vi "Constructor.vi"() -> ()   [LabVIEW 2015, in "IO Class.lvclass"]
uses:
  IO Class.lvclass
  Signal Settings.ctl
  Configuration.ctl
  Digital Indicator/Digital Indicator.lvclass
  Digital Control/Digital Control.lvclass
  Numeric Indicator/Numeric Indicator.lvclass
  Numeric Control/Numeric Control.lvclass
  FPGA Addon Input/FPGA Addon Input.lvclass
  FPGA Addon Output/FPGA Addon Output.lvclass
  IO Class.lvclass/IO Class.ctl
  EST Digital Event/Digital Event.lvclass
  EST Output/EST Output.lvclass
  EST Knock Sensor/EST Knock Sensor.lvclass
panel:
  out "IO Class.lvclass":refnum<class "IO Class.lvclass">
  out "error out":errorcluster
  in  "error in (no error)":errorcluster
  in  "Signal Settings":T1
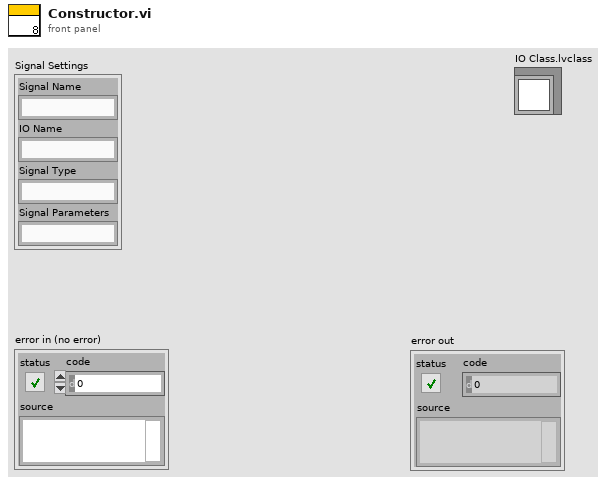
[diagram p1: front panel]
types:
  T1 = typedef "Signal Settings.ctl" = cluster{"Signal Name":string, "IO Name":string, "Signal Type":string, "Signal Parameters":string}
  T2 = typedef "Configuration.ctl" = cluster{"Classification":string, "Direction":string, "Type":string}
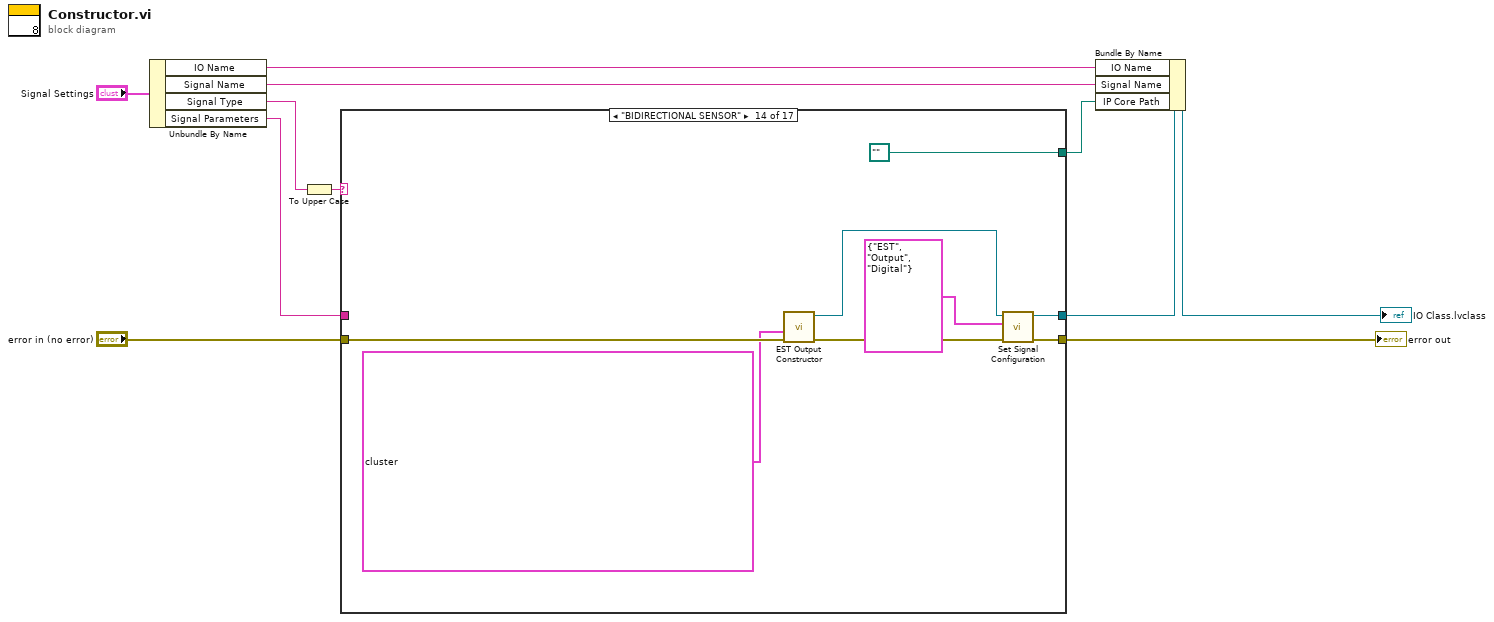
[diagram p0: block diagram]
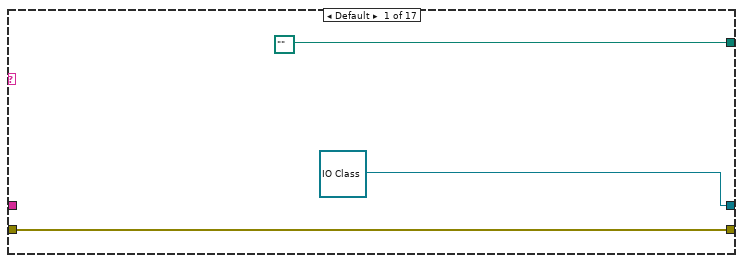
[diagram p2: hidden frame]
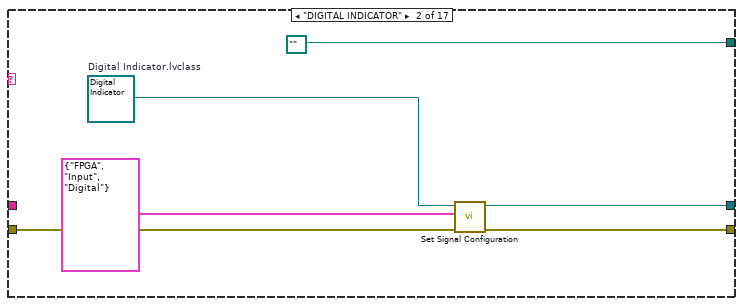
[diagram p3: hidden frame]
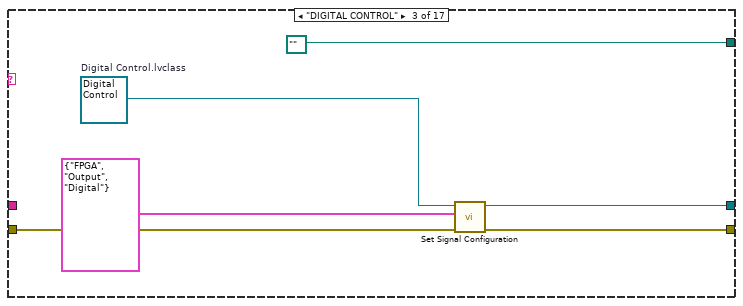
[diagram p4: hidden frame]
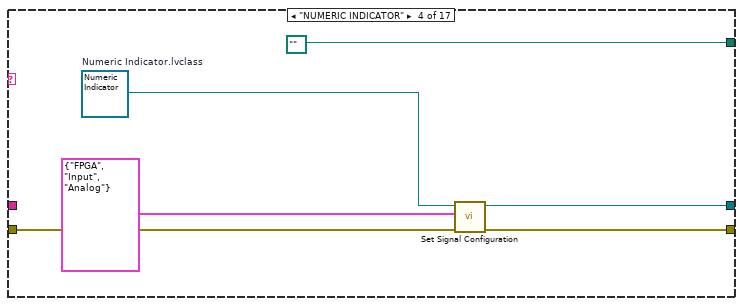
[diagram p5: hidden frame]
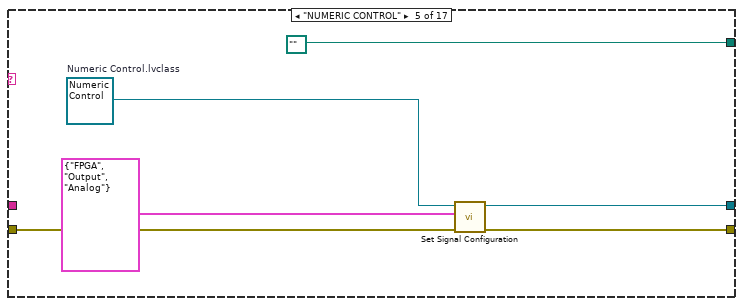
[diagram p6: hidden frame]
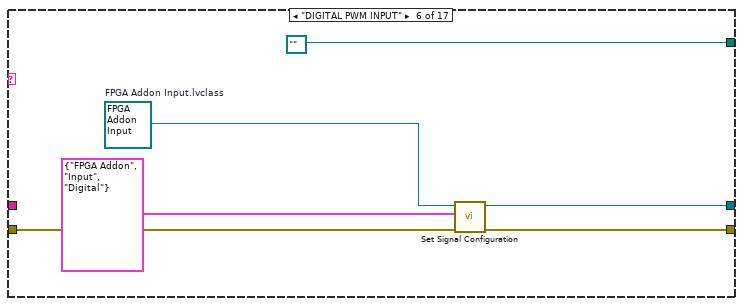
[diagram p7: hidden frame]
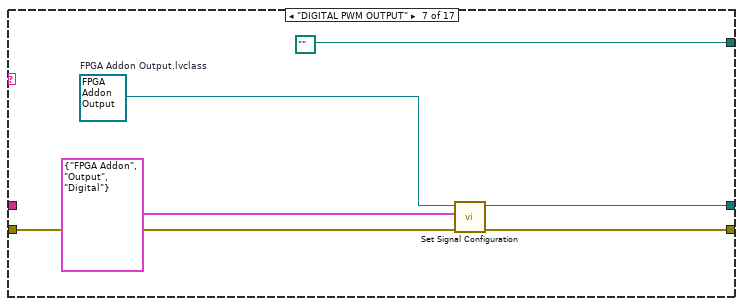
[diagram p8: hidden frame]
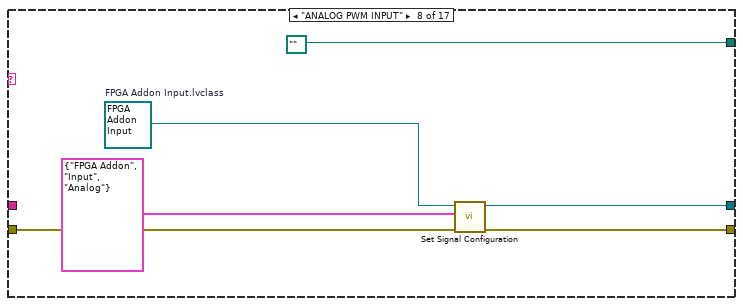
[diagram p9: hidden frame]
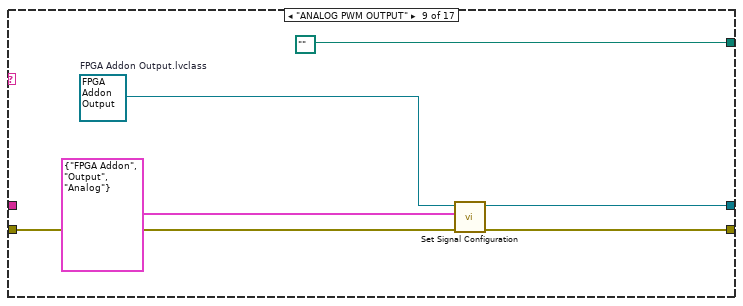
[diagram p10: hidden frame]
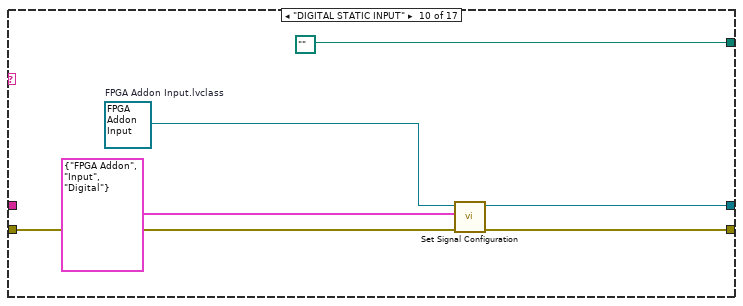
[diagram p11: hidden frame]
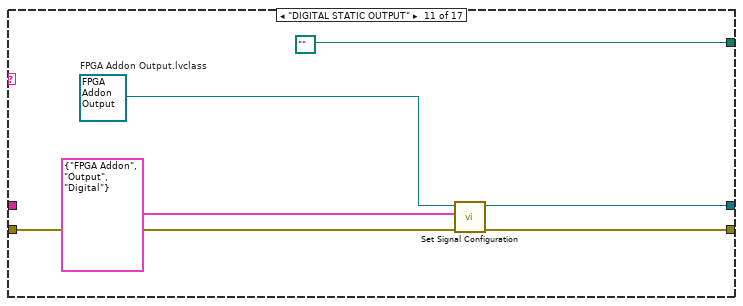
[diagram p12: hidden frame]
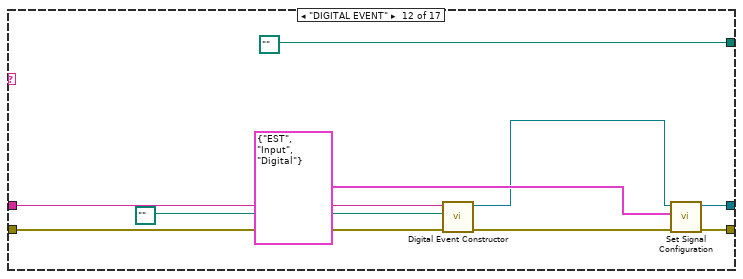
[diagram p13: hidden frame]
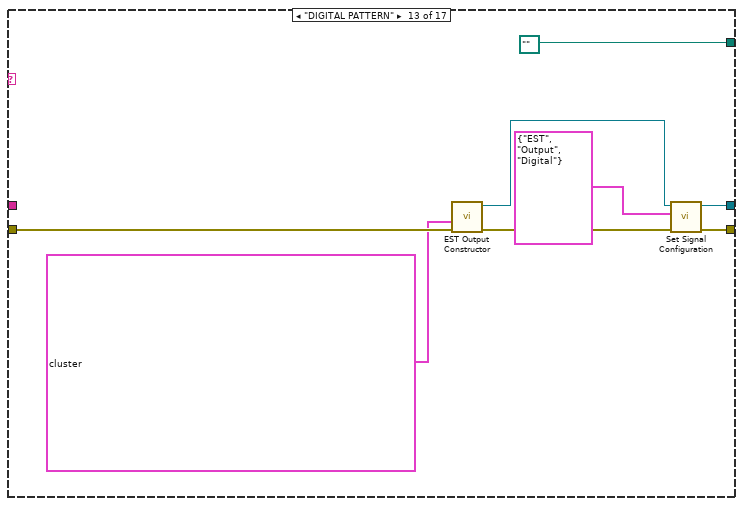
[diagram p14: hidden frame]
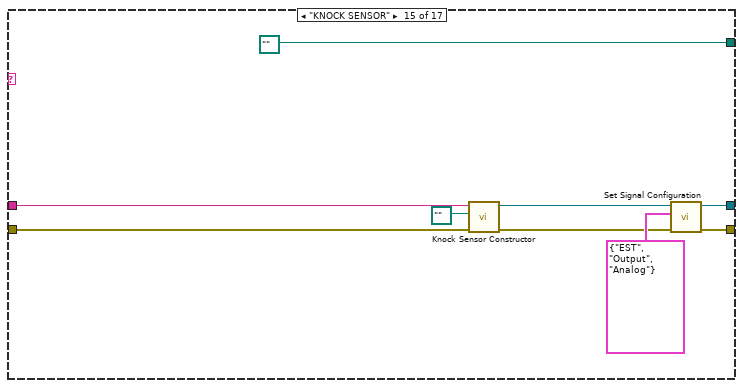
[diagram p15: hidden frame]
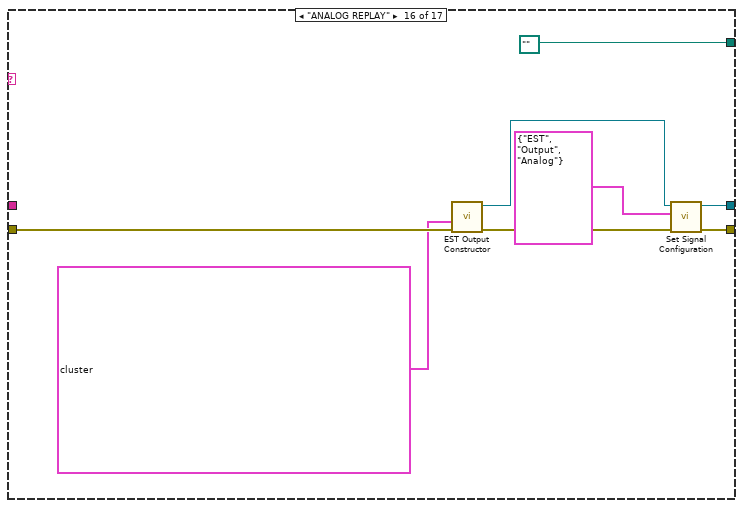
[diagram p16: hidden frame]
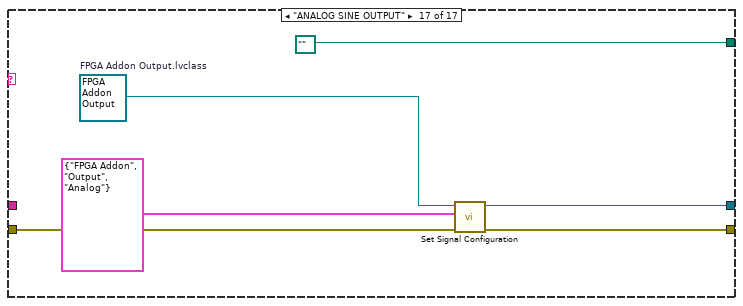
[diagram p17: hidden frame]
diagram:
  n1 = Unbundle By Name("Signal Settings") -> ("IO Name"=w5:string, "Signal Name"=w4:string, "Signal Type"=w10:string, "Signal Parameters"=w3:string)
  n2 = To Upper Case(1:w10) -> (0:w9:string)
  n3 = case shown="\"BIDIRECTIONAL SENSOR\"" w9 {
    tunnel: "error in (no error)" -> [w14 w20 w26 w32 w38 w43 w50 w55 w62 w67 w74 w79 w87 w95 w104 w112 w122]
    tunnel: [w14 w19 w25 w31 w37 w42 w49 w54 w61 w66 w73 w83 w91 w99 w108 w116 w121] -> w7
    tunnel: [refnum<class "IO Class.lvclass"> refnum ("IO Class.lvclass") w17 w23 w29 w35 w40 w47 w52 w59 w64 w71 w81 w89 w97 w106 w114 w119] -> w2
    tunnel: w3 -> [_ _ _ _ _ _ _ _ _ _ _ w80 _ _ w101 _ _]
    tunnel: [path "" path "" path "" path "" path "" path "" path "" path "" path "" path "" path "" path "" path "" path "" path "" path "" path ""] -> w1
    frame Default {
    }
    frame "DIGITAL INDICATOR" {
      w15 = refnum<class "Digital Indicator.lvclass"> refnum  # Digital Indicator.lvclass
      n4 = call "Set Signal Configuration.vi"("error in (no error)"=w20, "Configuration"=T2 {"Classification"="FPGA", "Direction"="Input", "Type"="Digital"}, "IO Class in"=w15) -> ("error out"=w19:errorcluster, "IO Class out"=w17:refnum<class "Digital Indicator.lvclass">)  [unwired: 7 in]
    }
    frame "DIGITAL CONTROL" {
      w21 = refnum<class "Digital Control.lvclass"> refnum  # Digital Control.lvclass
      n5 = call "Set Signal Configuration.vi"("error in (no error)"=w26, "Configuration"=T2 {"Classification"="FPGA", "Direction"="Output", "Type"="Digital"}, "IO Class in"=w21) -> ("error out"=w25:errorcluster, "IO Class out"=w23:refnum<class "Digital Control.lvclass">)  [unwired: 7 in]
    }
    frame "NUMERIC INDICATOR" {
      w27 = refnum<class "Numeric Indicator.lvclass"> refnum  # Numeric Indicator.lvclass
      n6 = call "Set Signal Configuration.vi"("error in (no error)"=w32, "Configuration"=T2 {"Classification"="FPGA", "Direction"="Input", "Type"="Analog"}, "IO Class in"=w27) -> ("error out"=w31:errorcluster, "IO Class out"=w29:refnum<class "Numeric Indicator.lvclass">)  [unwired: 7 in]
    }
    frame "NUMERIC CONTROL" {
      w33 = refnum<class "Numeric Control.lvclass"> refnum  # Numeric Control.lvclass
      n7 = call "Set Signal Configuration.vi"("error in (no error)"=w38, "Configuration"=T2 {"Classification"="FPGA", "Direction"="Output", "Type"="Analog"}, "IO Class in"=w33) -> ("error out"=w37:errorcluster, "IO Class out"=w35:refnum<class "Numeric Control.lvclass">)  [unwired: 7 in]
    }
    frame "DIGITAL PWM INPUT" {
      w44 = refnum<class "FPGA Addon Input.lvclass"> refnum  # FPGA Addon Input.lvclass
      n8 = call "Set Signal Configuration.vi"("error in (no error)"=w43, "Configuration"=T2 {"Classification"="FPGA Addon", "Direction"="Input", "Type"="Digital"}, "IO Class in"=w44) -> ("error out"=w42:errorcluster, "IO Class out"=w40:refnum<class "FPGA Addon Input.lvclass">)  [unwired: 7 in]
    }
    frame "DIGITAL PWM OUTPUT" {
      w45 = refnum<class "FPGA Addon Output.lvclass"> refnum  # FPGA Addon Output.lvclass
      n9 = call "Set Signal Configuration.vi"("error in (no error)"=w50, "Configuration"=T2 {"Classification"="FPGA Addon", "Direction"="Output", "Type"="Digital"}, "IO Class in"=w45) -> ("error out"=w49:errorcluster, "IO Class out"=w47:refnum<class "FPGA Addon Output.lvclass">)  [unwired: 7 in]
    }
    frame "ANALOG PWM INPUT" {
      w56 = refnum<class "FPGA Addon Input.lvclass"> refnum  # FPGA Addon Input.lvclass
      n10 = call "Set Signal Configuration.vi"("error in (no error)"=w55, "Configuration"=T2 {"Classification"="FPGA Addon", "Direction"="Input", "Type"="Analog"}, "IO Class in"=w56) -> ("error out"=w54:errorcluster, "IO Class out"=w52:refnum<class "FPGA Addon Input.lvclass">)  [unwired: 7 in]
    }
    frame "ANALOG PWM OUTPUT" {
      w57 = refnum<class "FPGA Addon Output.lvclass"> refnum  # FPGA Addon Output.lvclass
      n11 = call "Set Signal Configuration.vi"("error in (no error)"=w62, "Configuration"=T2 {"Classification"="FPGA Addon", "Direction"="Output", "Type"="Analog"}, "IO Class in"=w57) -> ("error out"=w61:errorcluster, "IO Class out"=w59:refnum<class "FPGA Addon Output.lvclass">)  [unwired: 7 in]
    }
    frame "DIGITAL STATIC INPUT" {
      w68 = refnum<class "FPGA Addon Input.lvclass"> refnum  # FPGA Addon Input.lvclass
      n12 = call "Set Signal Configuration.vi"("error in (no error)"=w67, "Configuration"=T2 {"Classification"="FPGA Addon", "Direction"="Input", "Type"="Digital"}, "IO Class in"=w68) -> ("error out"=w66:errorcluster, "IO Class out"=w64:refnum<class "FPGA Addon Input.lvclass">)  [unwired: 7 in]
    }
    frame "DIGITAL STATIC OUTPUT" {
      w69 = refnum<class "FPGA Addon Output.lvclass"> refnum  # FPGA Addon Output.lvclass
      n13 = call "Set Signal Configuration.vi"("error in (no error)"=w74, "Configuration"=T2 {"Classification"="FPGA Addon", "Direction"="Output", "Type"="Digital"}, "IO Class in"=w69) -> ("error out"=w73:errorcluster, "IO Class out"=w71:refnum<class "FPGA Addon Output.lvclass">)  [unwired: 7 in]
    }
    frame "DIGITAL EVENT" {
      n14 = call "Digital Event Constructor.vi"("error in (no error)"=w79, "Capture Path"=path "", "Signal Parameters"=w80) -> ("error out"=w78:errorcluster, "Digital Event.lvclass"=w77:refnum<class "Digital Event.lvclass">)  [unwired: 7 in]
      n15 = call "Set Signal Configuration.vi"("error in (no error)"=w78, "Configuration"=T2 {"Classification"="EST", "Direction"="Input", "Type"="Digital"}, "IO Class in"=w77) -> ("error out"=w83:errorcluster, "IO Class out"=w81:refnum<class "Digital Event.lvclass">)  [unwired: 7 in]
    }
    frame "DIGITAL PATTERN" {
      n16 = call "EST Output Constructor.vi"("error in (no error)"=w87, "Project Item"=cluster{"Name":string, "Value":variant}[] [{"Name"="FPGA.PersistentID", "Value"=variant(string "{CD7EB185-1A87-4E78-8C08-5D9A1491F439}")}, {"Name"="fullEmulation", "Value"=variant(bool TRUE)}, {"Name"="Memory Latency", "Value"=variant(u32 1)}, {"Name"="Multiple Clock Domains", "Value"=variant(bool FALSE)}, {"Name"="NI.LV.FPGA.CompileConfigString", "Value"=variant(string "Actual Number of Elements=1024;ReadArbs=2;WriteArbs=2;Implementation=2;DataType=100080000000000100094006000355313600010000000000000000;InitDataHash=;DRAM Selection=DramBank0;DRAM Max Outstanding Requests=64;DRAM Include Byte Enables=FALSE;DRAM Grant Time=50;Interface Configuration=Read A-Write B;Multiple Clock Domains=FALSE;Memory Latency=1")}, {"Name"="NI.LV.FPGA.MEMORY.ActualNumberOfElements", "Value"=variant(u32 1024)}, {"Name"="NI.LV.FPGA.MEMORY.DataWidth", "Value"=variant(u32 6)}, {"Name"="NI.LV.FPGA.MEMORY.DramIncludeByteEnables", "Value"=variant(bool FALSE)}, {"Name"="NI.LV.FPGA.MEMORY.DramMaxOutstandingRequests", "Value"=variant(i32 64)}, {"Name"="NI.LV.FPGA.MEMORY.DramSelection", "Value"=variant(string "DramBank0")}, {"Name"="NI.LV.FPGA.MEMORY.Init", "Value"=variant(bool FALSE)}, {"Name"="NI.LV.FPGA.MEMORY.InitData", "Value"=variant(string "")}, {"Name"="NI.LV.FPGA.MEMORY.InitVIPath", "Value"=variant(string "")}, {"Name"="NI.LV.FPGA.MEMORY.InterfaceAArbitration", "Value"=variant(u32 2)}, {"Name"="NI.LV.FPGA.MEMORY.InterfaceBArbitration", "Value"=variant(u32 2)}, {"Name"="NI.LV.FPGA.MEMORY.InterfaceConfig", "Value"=variant(u32 0)}, {"Name"="NI.LV.FPGA.MEMORY.RequestedNumberOfElements", "Value"=variant(u32 1024)}, {"Name"="NI.LV.FPGA.MEMORY.Type", "Value"=variant(u32 2)}, {"Name"="NI.LV.FPGA.ScriptConfigString", "Value"=variant(string "Actual Number of Elements=1024;ReadArbs=2;WriteArbs=2;Implementation=2;DataType=100080000000000100094006000355313600010000000000000000;InitDataHash=;DRAM Selection=DramBank0;DRAM Max Outstanding Requests=64;DRAM Include Byte Enables=FALSE;DRAM Grant Time=50;Interface Configuration=Read A-Write B;Multiple Clock Domains=FALSE;Memory Latency=1Persist Memory ValuesTRUE;")}, {"Name"="NI.LV.FPGA.Valid", "Value"=variant(bool TRUE)}, {"Name"="NI.LV.FPGA.Version", "Value"=variant(i32 10)}, {"Name"="Type Descriptor", "Value"=variant(string "100080000000000100094006000355313600010000000000000000")}] ("Array 2")) -> ("error out"=w86:errorcluster, "EST Output.lvclass"=w85:refnum<class "EST Output.lvclass">)  [unwired: 8 in]
      n17 = call "Set Signal Configuration.vi"("error in (no error)"=w86, "Configuration"=T2 {"Classification"="EST", "Direction"="Output", "Type"="Digital"}, "IO Class in"=w85) -> ("error out"=w91:errorcluster, "IO Class out"=w89:refnum<class "EST Output.lvclass">)  [unwired: 7 in]
    }
    frame "BIDIRECTIONAL SENSOR" {
      n18 = call "EST Output Constructor.vi"("error in (no error)"=w95, "Project Item"=cluster{"Name":string, "Value":variant}[] [{"Name"="FPGA.PersistentID", "Value"=variant(string "{CD7EB185-1A87-4E78-8C08-5D9A1491F439}")}, {"Name"="fullEmulation", "Value"=variant(bool TRUE)}, {"Name"="Memory Latency", "Value"=variant(u32 1)}, {"Name"="Multiple Clock Domains", "Value"=variant(bool FALSE)}, {"Name"="NI.LV.FPGA.CompileConfigString", "Value"=variant(string "Actual Number of Elements=1024;ReadArbs=2;WriteArbs=2;Implementation=2;DataType=100080000000000100094006000355313600010000000000000000;InitDataHash=;DRAM Selection=DramBank0;DRAM Max Outstanding Requests=64;DRAM Include Byte Enables=FALSE;DRAM Grant Time=50;Interface Configuration=Read A-Write B;Multiple Clock Domains=FALSE;Memory Latency=1")}, {"Name"="NI.LV.FPGA.MEMORY.ActualNumberOfElements", "Value"=variant(u32 1024)}, {"Name"="NI.LV.FPGA.MEMORY.DataWidth", "Value"=variant(u32 6)}, {"Name"="NI.LV.FPGA.MEMORY.DramIncludeByteEnables", "Value"=variant(bool FALSE)}, {"Name"="NI.LV.FPGA.MEMORY.DramMaxOutstandingRequests", "Value"=variant(i32 64)}, {"Name"="NI.LV.FPGA.MEMORY.DramSelection", "Value"=variant(string "DramBank0")}, {"Name"="NI.LV.FPGA.MEMORY.Init", "Value"=variant(bool FALSE)}, {"Name"="NI.LV.FPGA.MEMORY.InitData", "Value"=variant(string "")}, {"Name"="NI.LV.FPGA.MEMORY.InitVIPath", "Value"=variant(string "")}, {"Name"="NI.LV.FPGA.MEMORY.InterfaceAArbitration", "Value"=variant(u32 2)}, {"Name"="NI.LV.FPGA.MEMORY.InterfaceBArbitration", "Value"=variant(u32 2)}, {"Name"="NI.LV.FPGA.MEMORY.InterfaceConfig", "Value"=variant(u32 0)}, {"Name"="NI.LV.FPGA.MEMORY.RequestedNumberOfElements", "Value"=variant(u32 1024)}, {"Name"="NI.LV.FPGA.MEMORY.Type", "Value"=variant(u32 2)}, {"Name"="NI.LV.FPGA.ScriptConfigString", "Value"=variant(string "Actual Number of Elements=1024;ReadArbs=2;WriteArbs=2;Implementation=2;DataType=100080000000000100094006000355313600010000000000000000;InitDataHash=;DRAM Selection=DramBank0;DRAM Max Outstanding Requests=64;DRAM Include Byte Enables=FALSE;DRAM Grant Time=50;Interface Configuration=Read A-Write B;Multiple Clock Domains=FALSE;Memory Latency=1Persist Memory ValuesTRUE;")}, {"Name"="NI.LV.FPGA.Valid", "Value"=variant(bool TRUE)}, {"Name"="NI.LV.FPGA.Version", "Value"=variant(i32 10)}, {"Name"="Type Descriptor", "Value"=variant(string "100080000000000100094006000355313600010000000000000000")}] ("Array 2")) -> ("error out"=w94:errorcluster, "EST Output.lvclass"=w93:refnum<class "EST Output.lvclass">)  [unwired: 8 in]
      n19 = call "Set Signal Configuration.vi"("error in (no error)"=w94, "Configuration"=T2 {"Classification"="EST", "Direction"="Output", "Type"="Digital"}, "IO Class in"=w93) -> ("error out"=w99:errorcluster, "IO Class out"=w97:refnum<class "EST Output.lvclass">)  [unwired: 7 in]
    }
    frame "KNOCK SENSOR" {
      n20 = call "Knock Sensor Constructor.vi"("error in (no error)"=w104, "Generate Signal Path"=path "" ("Capture Path"), "Signal Parameters"=w101) -> ("error out"=w103:errorcluster, "EST Knock Sensor.lvclass"=w102:refnum<class "EST Knock Sensor.lvclass">)  [unwired: 7 in]
      n21 = call "Set Signal Configuration.vi"("error in (no error)"=w103, "Configuration"=T2 {"Classification"="EST", "Direction"="Output", "Type"="Analog"}, "IO Class in"=w102) -> ("error out"=w108:errorcluster, "IO Class out"=w106:refnum<class "EST Knock Sensor.lvclass">)  [unwired: 7 in]
    }
    frame "ANALOG REPLAY" {
      n22 = call "EST Output Constructor.vi"("error in (no error)"=w112, "Project Item"=cluster{"Name":string, "Value":variant}[] [{"Name"="FPGA.PersistentID", "Value"=variant(string "{CD7EB185-1A87-4E78-8C08-5D9A1491F439}")}, {"Name"="fullEmulation", "Value"=variant(bool TRUE)}, {"Name"="Memory Latency", "Value"=variant(u32 1)}, {"Name"="Multiple Clock Domains", "Value"=variant(bool FALSE)}, {"Name"="NI.LV.FPGA.CompileConfigString", "Value"=variant(string "Actual Number of Elements=16384;ReadArbs=2;WriteArbs=2;Implementation=2;DataType=100080000000000100094002000349313600010000000000000000;InitDataHash=;DRAM Selection=DramBank0;DRAM Max Outstanding Requests=64;DRAM Include Byte Enables=FALSE;DRAM Grant Time=50;Interface Configuration=Read A-Write B;Multiple Clock Domains=FALSE;Memory Latency=1")}, {"Name"="NI.LV.FPGA.MEMORY.ActualNumberOfElements", "Value"=variant(u32 16384)}, {"Name"="NI.LV.FPGA.MEMORY.DataWidth", "Value"=variant(u32 2)}, {"Name"="NI.LV.FPGA.MEMORY.DramIncludeByteEnables", "Value"=variant(bool FALSE)}, {"Name"="NI.LV.FPGA.MEMORY.DramMaxOutstandingRequests", "Value"=variant(i32 64)}, {"Name"="NI.LV.FPGA.MEMORY.DramSelection", "Value"=variant(string "DramBank0")}, {"Name"="NI.LV.FPGA.MEMORY.Init", "Value"=variant(bool FALSE)}, {"Name"="NI.LV.FPGA.MEMORY.InitData", "Value"=variant(string "")}, {"Name"="NI.LV.FPGA.MEMORY.InitVIPath", "Value"=variant(string "")}, {"Name"="NI.LV.FPGA.MEMORY.InterfaceAArbitration", "Value"=variant(u32 2)}, {"Name"="NI.LV.FPGA.MEMORY.InterfaceBArbitration", "Value"=variant(u32 2)}, {"Name"="NI.LV.FPGA.MEMORY.InterfaceConfig", "Value"=variant(u32 0)}, {"Name"="NI.LV.FPGA.MEMORY.RequestedNumberOfElements", "Value"=variant(u32 16384)}, {"Name"="NI.LV.FPGA.MEMORY.Type", "Value"=variant(u32 2)}, {"Name"="NI.LV.FPGA.ScriptConfigString", "Value"=variant(string "Actual Number of Elements=16384;ReadArbs=2;WriteArbs=2;Implementation=2;DataType=100080000000000100094002000349313600010000000000000000;InitDataHash=;DRAM Selection=DramBank0;DRAM Max Outstanding Requests=64;DRAM Include Byte Enables=FALSE;DRAM Grant Time=50;Interface Configuration=Read A-Write B;Multiple Clock Domains=FALSE;Memory Latency=1Persist Memory ValuesTRUE;")}, {"Name"="NI.LV.FPGA.Valid", "Value"=variant(bool TRUE)}, {"Name"="NI.LV.FPGA.Version", "Value"=variant(i32 10)}, {"Name"="Type Descriptor", "Value"=variant(string "100080000000000100094002000349313600010000000000000000")}] ("Array 2")) -> ("error out"=w111:errorcluster, "EST Output.lvclass"=w110:refnum<class "EST Output.lvclass">)  [unwired: 8 in]
      n23 = call "Set Signal Configuration.vi"("error in (no error)"=w111, "Configuration"=T2 {"Classification"="EST", "Direction"="Output", "Type"="Analog"}, "IO Class in"=w110) -> ("error out"=w116:errorcluster, "IO Class out"=w114:refnum<class "EST Output.lvclass">)  [unwired: 7 in]
    }
    frame "ANALOG SINE OUTPUT" {
      w117 = refnum<class "FPGA Addon Output.lvclass"> refnum  # FPGA Addon Output.lvclass
      n24 = call "Set Signal Configuration.vi"("error in (no error)"=w122, "Configuration"=T2 {"Classification"="FPGA Addon", "Direction"="Output", "Type"="Analog"}, "IO Class in"=w117) -> ("error out"=w121:errorcluster, "IO Class out"=w119:refnum<class "FPGA Addon Output.lvclass">)  [unwired: 7 in]
    }
  }
  "error out" <- w7
  n25 = Bundle By Name(cluster=w2, "IO Name"=w5, "Signal Name"=w4, "IP Core Path"=w1) -> (→"IO Class.lvclass":refnum<class "IO Class.lvclass">)
